vi "acquisition.vi"() -> ()   [LabVIEW 2013]
panel:
  out "signal 2":dynamicdata(graph)
  out "Signal 1":dynamicdata(graph)
  in  "particle?":bool caption="particle"
  out "red = signal 2, white = signal 1":dynamicdata(graph)
  in  "stop (F)":bool
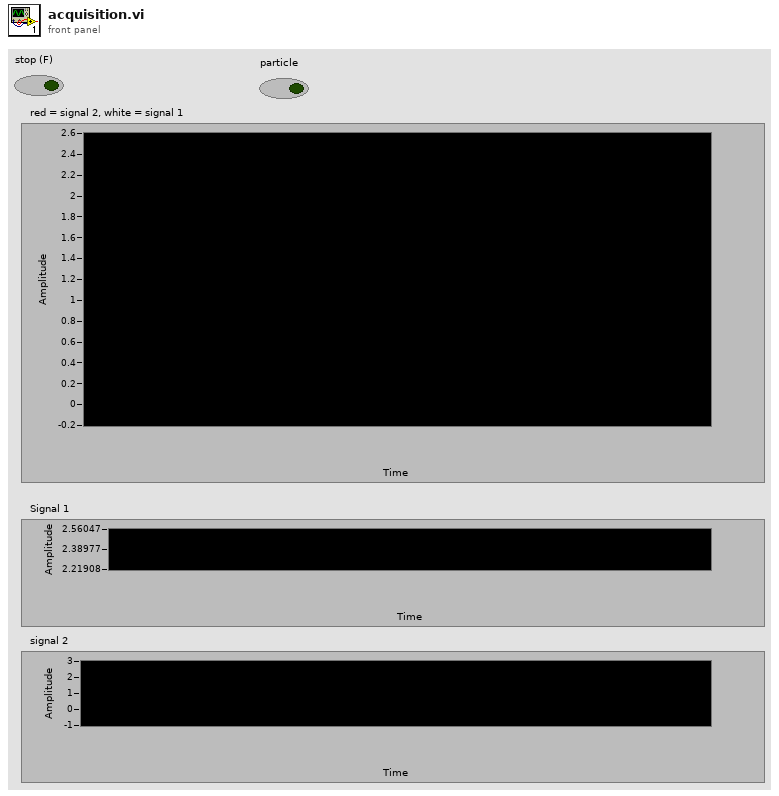
[diagram p1: front panel]
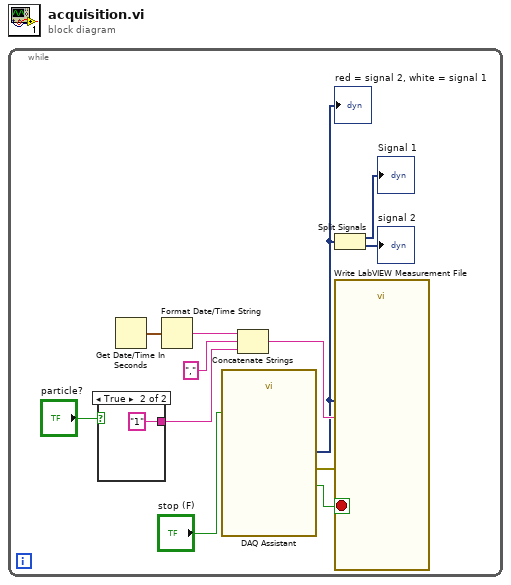
[diagram p0: block diagram]
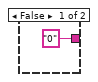
[diagram p2: hidden frame]
diagram:
  n1 = while {
    stop <- w11 stop-if-true
    n2 = case shown="True" "particle?" {
      tunnel: ["0" "1"] -> w5
      frame False {
      }
      frame True {
      }
    }
    n3 = Get Date/Time In Seconds() -> (seconds since 1Jan1904=w10:timestamp)
    n4 = Format Date/Time String(seconds (now)=w10) -> (date/time string=w9:string)  [unwired: 2 in]
    n5 = call "DAQ Assistant"("stop (F)"="stop (F)") -> ("data"=w3:dynamicdata, "stopped"=w11:bool, "error out"=w7:errorcluster)  [unwired: 15 in, 1 out]
    "red = signal 2, white = signal 1" <- w3
    n6 = Concatenate Strings(w9, ",", w5) -> (w8:string)
    n7 = Split Signals(w3) -> (→"Signal 1":dynamicdata, →"signal 2":dynamicdata)  [unwired: 2 in]
    n8 = call "Write LabVIEW Measurement File"("Signals"=w3, "error in (no error)"=w7, "Comment"=w8) -> ()  [unwired: 14 in, 3 out]
  }
